vi "Release.vi"(7 "Formatter (Default)":refnum<class "MultiError Formatter.lvclass">, 10 "MultiErrors in":refnum<class "MultiErrors.lvclass">, 11 "Upstream Error (None)":errorcluster) -> (2 "error out":errorcluster)   [LabVIEW 2020, in "VolatusErrorUtilities.lvlib" / "MultiErrors.lvclass"]
uses:
  MultiErrors.lvclass
  MultiError Formatter/MultiError Formatter.lvclass
  MultiErrors.lvclass/MultiErrors.ctl
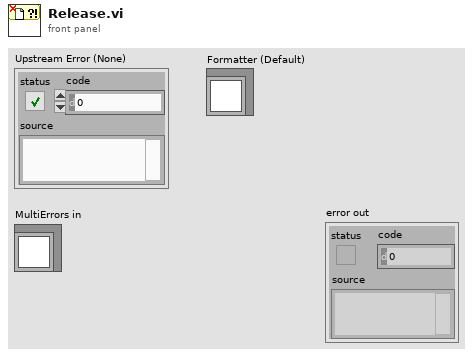
[diagram p1: front panel]
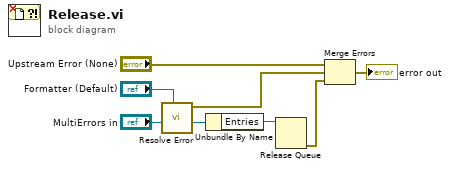
[diagram p0: block diagram]
diagram:
  n1 = call "Resolve Error.vi"("Formatter (Default)"="Formatter (Default)", "MultiErrors in"="MultiErrors in") -> ("MultiErrors out"=w3:refnum<class "MultiErrors.lvclass">, "error out"=w4:errorcluster)  [unwired: 8 in]
  n2 = Unbundle By Name(w3) -> ("Entries"=w8:refnum<queue>)
  n3 = Release Queue(queue=w8) -> (error out=w5:errorcluster)  [unwired: 2 in, 2 out]
  n4 = Merge Errors("Upstream Error (None)", w4, w5) -> (→"error out":errorcluster)
